vi "GetUIStateChangeEvents.vi"(8 "error in (no error)":errorcluster, 11 "SMO.UI.MAUI in":refnum<class "SMO.UI.MAUI.lvclass">) -> (0 "error out":errorcluster, 2 "UI State Change":refnum<user-event>[](array[refnum]), 3 "SMO.UI.MAUI out":refnum<class "SMO.UI.MAUI.lvclass">)   [LabVIEW 2016, in "SMO.UI.MAUI.lvclass"]
uses:
  SMO.UI.MAUI.lvclass
  <vilib>/Levylab/SMO.UI.Embedded/Typedefs/UI State.ctl
  <vilib>/JKI/JKI SMO/SMO/SMO.lvclass
  SMO.UI.MAUI.lvclass/SMO.UI.MAUI.ctl
  <vilib>/Levylab/SMO.UI.Embedded/SMO.UI.Embedded.lvclass
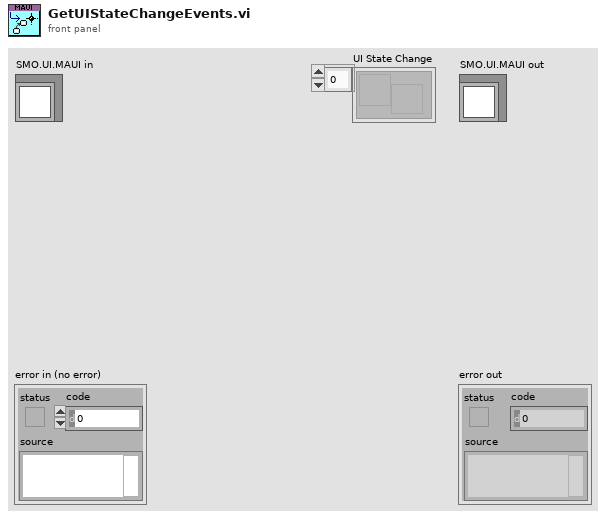
[diagram p1: front panel]
types:
  T1 = typedef "SMO.UI.Embedded.lvclass/PublicEvents--Cluster.ctl" = cluster{"ReadyForInfo":refnum<user-event>, "UIStateChange":refnum<user-event>}
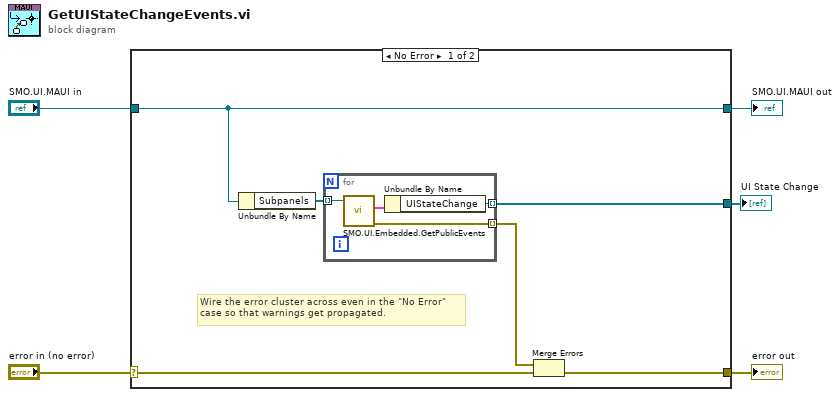
[diagram p0: block diagram]
diagram:
  n1 = case shown="No Error" "error in (no error)" {
    selector: "error in (no error)" -> [w8 w17]
    tunnel: [w6 w17] -> w4
    tunnel: [w10 w16] -> w2
    tunnel: "SMO.UI.MAUI in" -> [w10 w16]
    tunnel: [w7 _] -> w1
    frame No Error {
      # "Wire the error cluster across even in the \"No Error\"\ncase so that warnings get propagated."
      n2 = Unbundle By Name(w10) -> ("Subpanels"=w11:refnum<class "SMO.UI.Embedded.lvclass">[])
      n3 = for {
        tunnel: w11 -> [w15] mode=indexing
        tunnel: [w13] -> w7 mode=indexing
        tunnel: [w12] -> w9 mode=indexing
        n4 = call <vilib>:"SMO.UI.Embedded.GetPublicEvents.vi"("EmbeddedSMO"=w15) -> ("error out"=w12:errorcluster, "Public Events"=w14:T1)  [unwired: 8 in, 1 out]
        n5 = Unbundle By Name(w14) -> ("UIStateChange"=w13:refnum<user-event>)
      }
      n6 = Merge Errors(w9, w8) -> (w6:errorcluster)
    }
    frame Error {
    }
  }
  "error out" <- w4
  "SMO.UI.MAUI out" <- w2
  "UI State Change" <- w1
